vi "conversion_interpolation.vi"() -> ()   [LabVIEW 2013]
uses:
  <vilib>/gmath/NI_Gmath.lvlib
panel:
  out "yi":dbl[](array[numeric]) format="%_6g"
  in  "xi":dbl[](array[numeric]) format="%_6g"
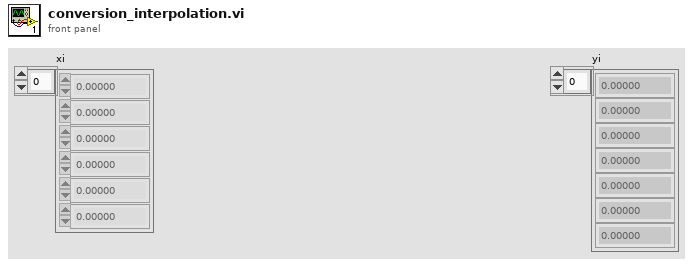
[diagram p1: front panel]
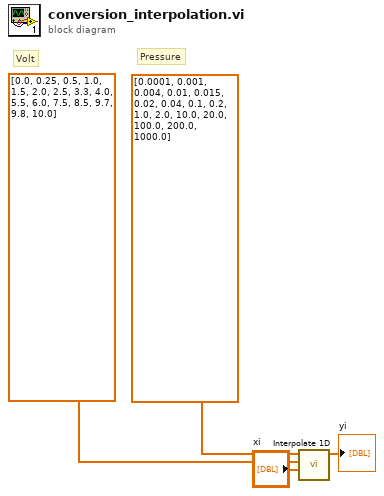
[diagram p0: block diagram]
diagram:
  # "Pressure"
  # "Volt"
  n1 = call <vilib>:"Interpolate 1D.vi"("xi"="xi", "X"=dbl[] [0.0, 0.25, 0.5, 1.0, 1.5, 2.0, 2.5, 3.3, 4.0, 5.5, 6.0, 7.5, 8.5, 9.7, 9.8, 10.0] ("Y"), "Y"=dbl[] [0.0001, 0.001, 0.004, 0.01, 0.015, 0.02, 0.04, 0.1, 0.2, 1.0, 2.0, 10.0, 20.0, 100.0, 200.0, 1000.0]) -> ("yi"=→"yi":dbl[])  [unwired: 6 in, 2 out]
